vi "FiberSpectrograph_getEvent_internalCommand.vi"(8 "error in (no error)":errorcluster, 11 "logevent_internalCommand_Ctl":T1) -> (0 "error out":errorcluster, 2 "function return":i32, 3 "logevent_internalCommand_Ctl out":T1)   [LabVIEW 2016, in "SALLV_FiberSpectrograph.lvlib"]
doc: "int FiberSpectrograph_shm_getEvent_internalCommandLV(FiberSpectrograph_logevent_internalCommandLV *logevent_internalCommand_Ctl );"
uses:
  SALLV_FiberSpectrograph.lvlib
  DataTypes/logevent_internalCommand.ctl
  SALLV_FiberSpectrograph.so
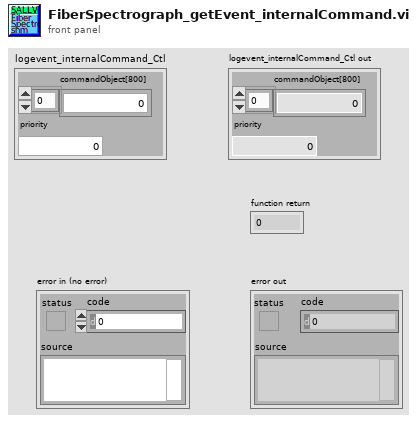
[diagram p1: front panel]
types:
  T1 = typedef "SALLV_FiberSpectrograph.lvlib/logevent_internalCommand.ctl" = cluster{"commandObject[800]":u8[], "priority":i32}
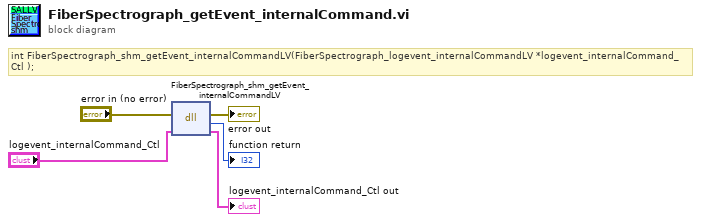
[diagram p0: block diagram]
diagram:
  # "int FiberSpectrograph_shm_getEvent_internalCommandLV(FiberSpectrograph_logevent_internalCommandLV *logevent_internalCommand_Ctl );"
  n1 = dll-call lib="home/harini/Documents/lsst/SALLV_FiberSpectrograph/SALLV_FiberSpectrograph.*" fn="FiberSpectrograph_shm_getEvent_internalCommandLV"(error in="error in (no error)", "logevent_internalCommand_Ctl"="logevent_internalCommand_Ctl") -> (error out=→"error out":errorcluster, →"function return":i32, "logevent_internalCommand_Ctl"=→"logevent_internalCommand_Ctl out":T1)  [unwired: 2 in, 1 out]
